vi "Read Host Stream.vi"(4 "XNET Frames":refnum<queue>, 5 "Host Parameters":T1, 6 "Log":bool, 7 "Init?":bool, 8 "error in (no error)":errorcluster, 11 "Refs in":T6) -> (0 "error out":errorcluster, 2 "Stream":T5, 3 "Refs out":T6)   [LabVIEW 2019, in "CAN Stream Support Workspace Shared.lvlib"]
uses:
  CAN Stream Support Workspace Shared.lvlib
  Types/Host Stream Refs.ctl
  <vilib>/xnet/xnet.llb/XNET CAN Comm.ctl
  <vilib>/xnet/xnet.llb/XNET CAN Comm State.ctl
  <vilib>/xnet/xnet.llb/XNET CAN Last Err.ctl
  <vilib>/xnet/xnet.llb/XNET Frame CAN.ctl
  <vilib>/xnet/xnet.llb/XNET Frame Type CAN.ctl
  Types/Host Stream Data.ctl
  Types/Host Stream Engine Parameters.ctl
  Addon/Addon Shared/Types/Filter Parameters.ctl
  Addon/Addon Shared/Types/Direction Filter.ctl
  Addon/Addon Shared/Types/Type Filter.ctl
  Convert Frame Array to String Array.vi
  <vilib>/dlg_ctls.llb/Space Constant.vi
  <vilib>/Utility/error.llb/Trim Whitespace.vi
  Convert Time to UTC String.vi
  <vilib>/Utility/error.llb/Trim Whitespace One-Sided.vi
  <userlib>/_OpenG.lib/array/array.llb/Sort Array__ogtk.vi
  <userlib>/_OpenG.lib/array/array.llb/Sort 2D Array (String)__ogtk.vi
  <resource>/objmgr/ni.dex.rc
  Addon/Addon Shared/CAN Stream Support Shared.lvlib
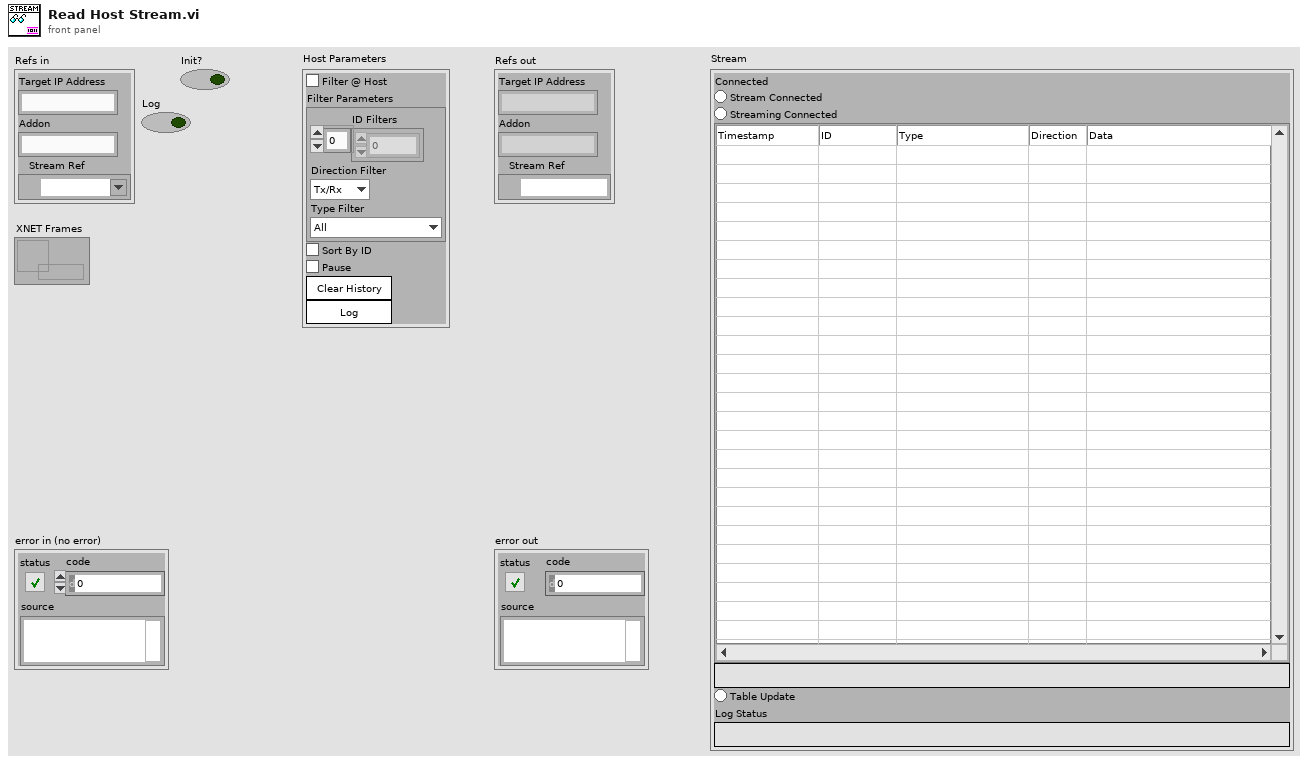
[diagram p1: front panel]
types:
  T1 = typedef "CAN Stream Support Workspace Shared.lvlib/Host Stream Engine Parameters.ctl" = cluster{"Host Filter":bool, "Filter Parameters":T2, "Sort By ID":bool, "Pause":bool, "Clear History":bool, "Log":bool}
  T2 = typedef "CAN Stream Support Shared.lvlib/Filter Parameters.ctl" = cluster{"ID Filters":u32[], "Direction Filter":T3, "Type Filter":T4}
  T3 = typedef "CAN Stream Support Shared.lvlib/Direction Filter.ctl" = enum16{"Tx/Rx", "Rx", "Tx"}
  T4 = typedef "CAN Stream Support Shared.lvlib/Type Filter.ctl" = enum16{"All", "CAN Data", "CAN Remote", "CAN Bus Error", "CAN 2.0 Data", "CAN FD Data", "CAN FD+BRS Data", "J1939 Data", "Delay", "Log Trigger", "Start Trigger"}
  T5 = typedef "CAN Stream Support Workspace Shared.lvlib/Host Stream Data.ctl" = cluster{"Connected":bool, "Bus Data Update":bool, "Bus Data":string[][], "Bus Status":string, "Bus Warning":bool, "Log Status":string}
  T6 = typedef "CAN Stream Support Workspace Shared.lvlib/Host Stream Refs.ctl" = cluster{"Target IP Address":string, "Addon":string, "Stream Ref":refnum<k21>}
  T7 = typedef "XNET CAN Comm.ctl" = cluster{"fault code":i32, "fault?":bool, "communication state":T8, "last error":T9, "receive error counter":u8, "transmit error counter":u8, "transceiver error?":bool, "sleep?":bool}
  T8 = typedef "XNET CAN Comm State.ctl" = u8
  T9 = typedef "XNET CAN Last Err.ctl" = u8
  T10 = typedef "XNET Frame CAN.ctl" = cluster{"timestamp":timestamp, "payload":u8[], "identifier":u32, "type":T11, "extended?":bool, "echo?":bool}
  T11 = typedef "XNET Frame Type CAN.ctl" = u8
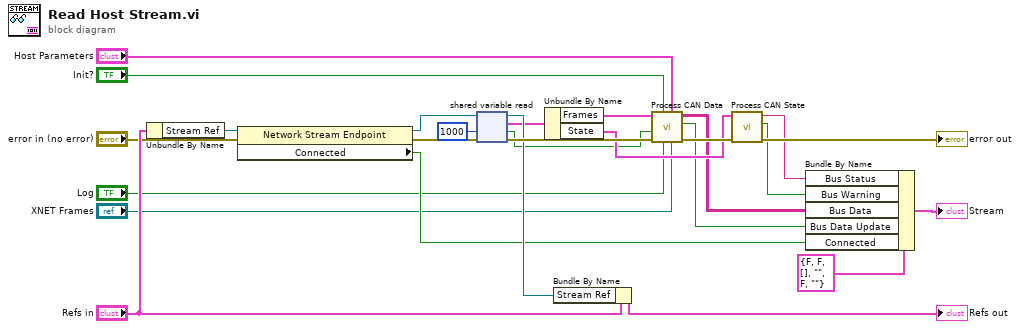
[diagram p0: block diagram]
diagram:
  n1 = Unbundle By Name("Refs in") -> ("Stream Ref"=w21:refnum<k21>)
  n2 = property class="Network Stream Endpoint"(reference=w21, error in="error in (no error)") -> (reference out=w18:refnum<k21>, error out=w20:errorcluster, "Connected"=w8:bool)
  n3 = shared-variable-read(w18, w20, 1000 ("timeout ms")) -> (w23:refnum<k21>, w25:errorcluster, w5:bool, w14:cluster{"State":T7, "Frames":T10[]})
  n4 = Unbundle By Name(w14) -> ("Frames"=w6:T10[], "State"=w13:T7)
  n5 = Bundle By Name(cluster="Refs in", "Stream Ref"=w23) -> (→"Refs out":T6)
  n6 = call "Process CAN Data.vi"("XNET Frames"="XNET Frames", "Host Parameters"="Host Parameters", "Log"="Log", "Init?"="Init?", "error in (no error)"=w25, "Data Timed Out?"=w5, "Data"=w6) -> ("error out"=w16:errorcluster, "Table Update"=w4:bool, "Table"=w7:string[][])  [unwired: 2 in]
  n7 = call "Process CAN State.vi"("error in (no error)"=w16, "State"=w13) -> ("error out"=→"error out":errorcluster, "Warning"=w9:bool, "State"=w10:string)  [unwired: 7 in]
  n8 = Bundle By Name(cluster=T5 {"Connected"=FALSE, "Bus Data Update"=FALSE, "Bus Data"=[], "Bus Status"="", "Bus Warning"=FALSE, "Log Status"=""} ("Stream"), "Bus Status"=w10, "Bus Warning"=w9, "Bus Data"=w7, "Bus Data Update"=w4, "Connected"=w8) -> (→"Stream":T5)
